vi "Populate Subpanels.vi"(8 "error in (no error)":errorcluster, 9 "View Labels (optional)":string[](array[string]), 10 "Views":refnum<class "Message Enqueuer.lvclass">[](array[class]), 11 "IViewModel In":refnum<class "IViewModel.lvclass">) -> (0 "error out":errorcluster, 3 "IViewModel Out":refnum<class "IViewModel.lvclass">)   [LabVIEW 2015, in "IViewModel.lvlib" / "IViewModel.lvclass"]
doc: "<License>\nCopyright © 2017 Composed Systems, LLC | All rights reserved\nwww.composed.io\n\nAuthor: Ethan Stern <ethan.stern@composed.io>\n\nThis software is provided \"AS IS\" WITHOUT WARRANTIES, either express or implied, AND IS FOR EDUCATIONAL PURPOSES ONLY.\n</License>"
uses:
  IViewModel.lvclass
  <vilib>/ActorFramework/Message Enqueuer/Message Enqueuer.lvclass
  IViewModel.lvclass/IViewModel.ctl
  IViewable/IViewable Messages/Insert Front Panel Msg/Insert Front Panel Msg.lvclass/Insert Front Panel Msg.ctl
  <vilib>/ActorFramework/Message Enqueuer/Message Enqueuer.lvclass/Message Enqueuer.ctl
  <vilib>/ActorFramework/Message Enqueuer/Enqueue.vi
  <vilib>/ActorFramework/Message Priority Queue/Priority Enqueue.vi
  IViewManager/IViewManager/IViewManager.lvclass
  IViewable/IViewable Messages/Insert Front Panel Msg/Insert Front Panel Msg.lvclass
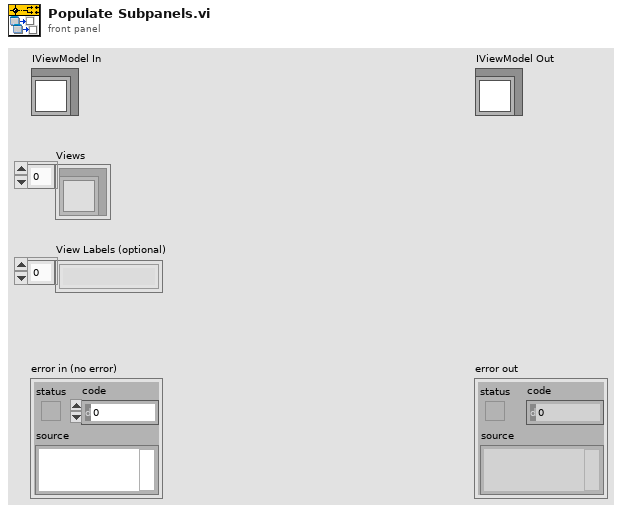
[diagram p1: front panel]
types:
  T1 = typedef "IViewable.lvlib/ProtectedSubpanel.lvclass/Protected Subpanel Reference.ctl" = refnum<data-value>
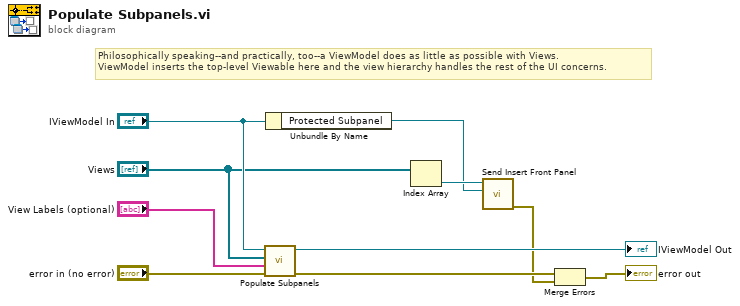
[diagram p0: block diagram]
diagram:
  # "Philosophically speaking--and practically, too--a ViewModel does as little as possible with Views.\nViewModel inserts the top-level Viewable here and the view hierarchy handles the rest of the UI concerns."
  n1 = call-parent "Populate Subpanels.vi"("error in (no error)"="error in (no error)", "View Labels (optional)"="View Labels (optional)", "Views"="Views", "IViewManager In"="IViewModel In") -> ("error out"=w10:errorcluster, "IViewManager Out"=→"IViewModel Out":refnum<class "IViewModel.lvclass">)  [unwired: 6 in]
  n2 = Unbundle By Name("IViewModel In") -> ("Protected Subpanel"=w4:T1)
  n3 = Index Array(array="Views") -> (element=w5:refnum<class "Message Enqueuer.lvclass">)  [unwired: 1 in]
  n4 = call "Send Insert Front Panel.vi"("Protected Subpanel"=w4, "Message Enqueuer"=w5) -> ("error out"=w2:errorcluster)  [unwired: 8 in, 1 out]
  n5 = Merge Errors(w10, w2) -> (→"error out":errorcluster)
